vi "_TBD Constant - Date-Time Format Code String.vi"() -> (0 "Date-Time Format String":string="%Y-%m-%d %H_%M_%S")   [LabVIEW 2023, in "Error Manager.lvlib" / "Error Log.lvclass"]
uses:
  Error Log.lvclass
  Error Log.lvclass/Error Log.ctl
panel:
  # "Input\nInputs to the VI"
  # "Development\nControls or indicators that are useful for development or testing, but which are not outputs of the VI."
  # "Output\nOutputs of the VI"
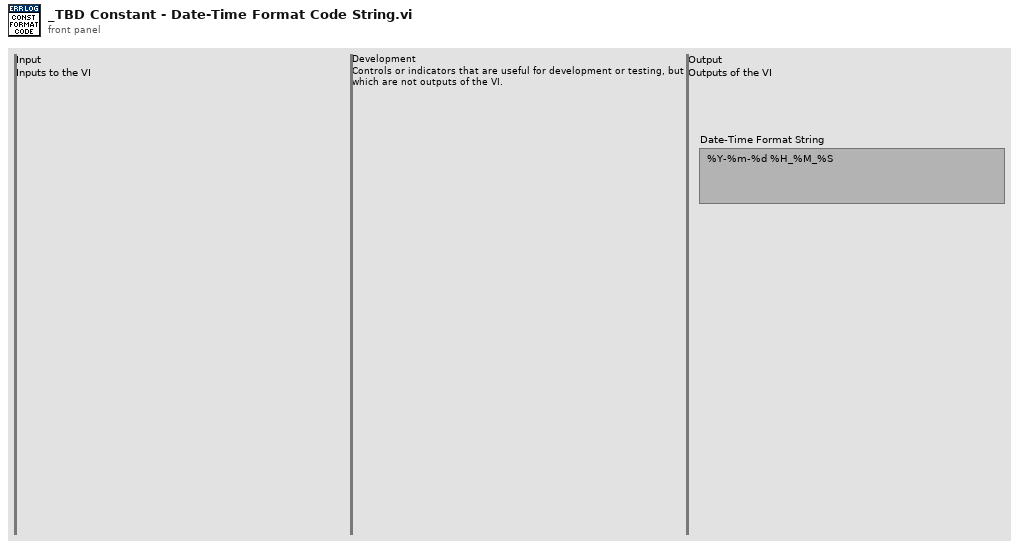
[diagram p1: front panel]
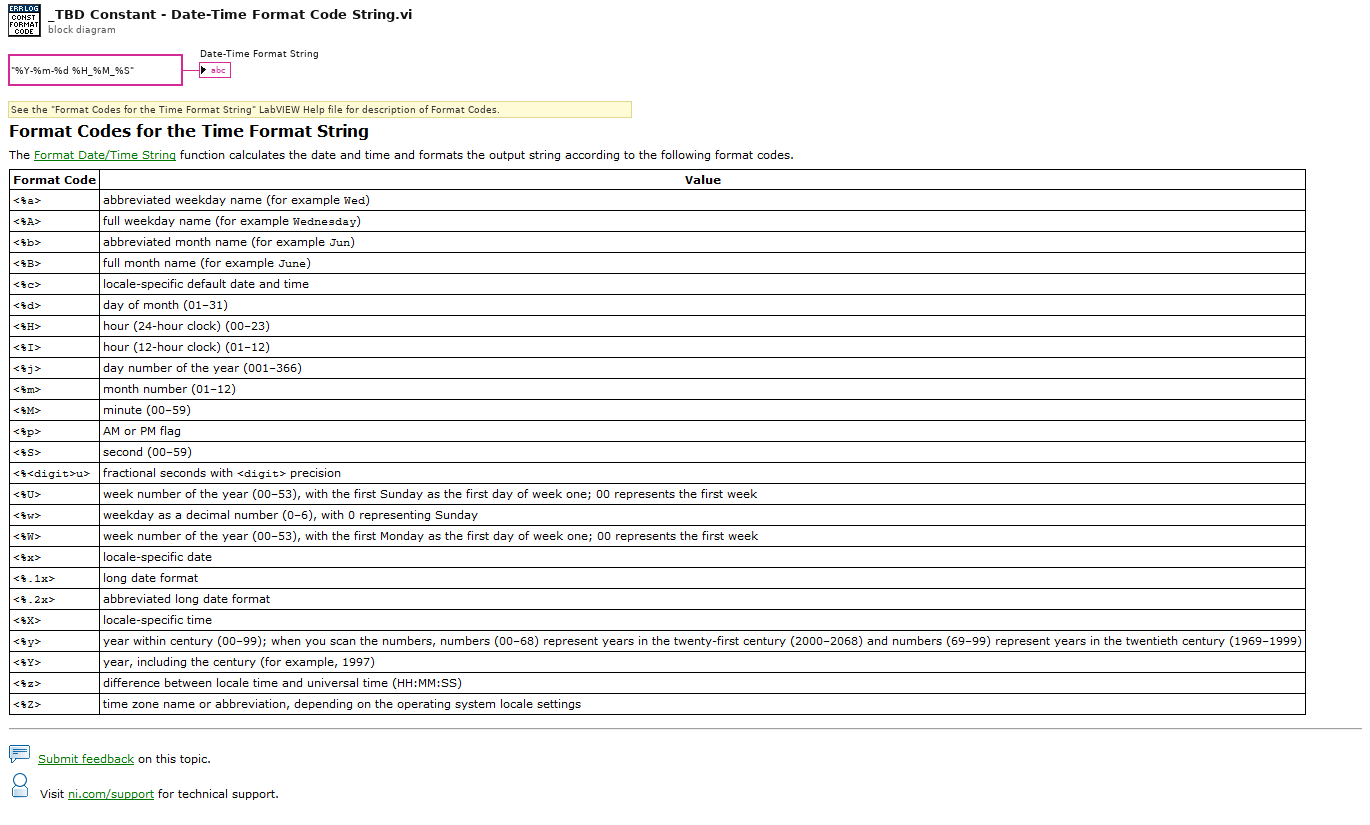
[diagram p0: block diagram]
diagram:
  # "See the \"Format Codes for the Time Format String\" LabVIEW Help file for description of Format Codes."
  "Date-Time Format String" <- "%Y-%m-%d %H_%M_%S" ("time format string (%c)")
